vi "CMD_GETFLOATPOPUP.vi"(6 "Gantry in":refnum<class "Gantry.lvclass">, 8 "error in (no error)":errorcluster, 10 "Arguments":string[](array[string]), 11 "gScript Interpreter in":refnum<class "gScript Interpreter.lvclass">) -> (0 "error out":errorcluster, 3 "gScript Interpreter out":refnum<class "gScript Interpreter.lvclass">, 4 "Gantry out":refnum<class "Gantry.lvclass">)   [LabVIEW 2022 SP3, in "gScript Interpreter.lvclass"]
uses:
  gScript Interpreter.lvclass
  gScript Interpreter.lvclass/gScript Interpreter.ctl
  Shared Components/Gantry Class/Gantry.lvclass
panel:
  out "Message":string
  in  "Input":dbl format="%#g"
  in  "OK":bool caption="OK1"
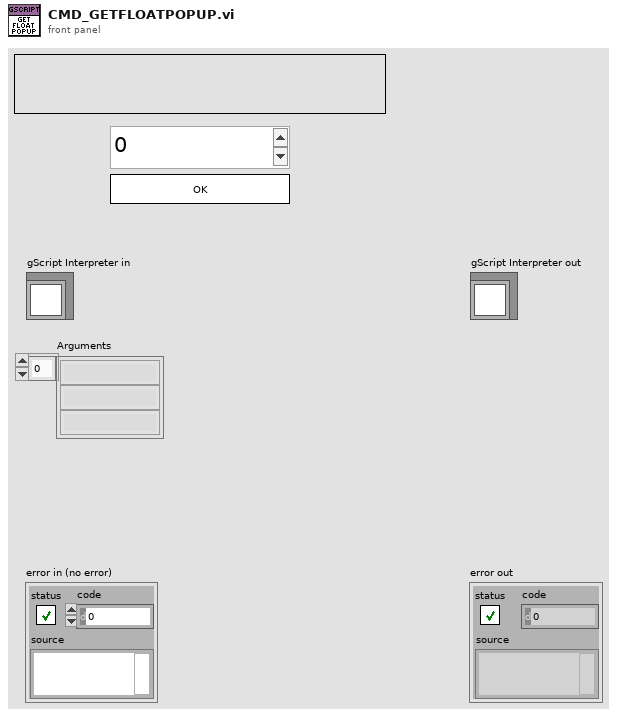
[diagram p1: front panel]
types:
  T1 = typedef "Memory Cell.ctl" = cluster{"type":T2, "x":dbl, "y":dbl, "z":dbl, "w":dbl}
  T2 = typedef "Memory Cell Type Enum.ctl" = enum16{"integer", "float", "vector", "rotation"}
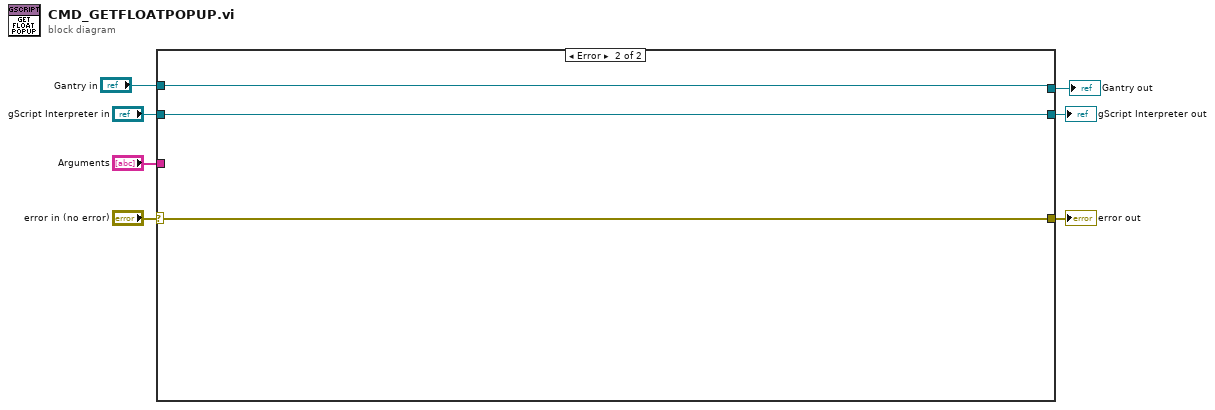
[diagram p0: block diagram]
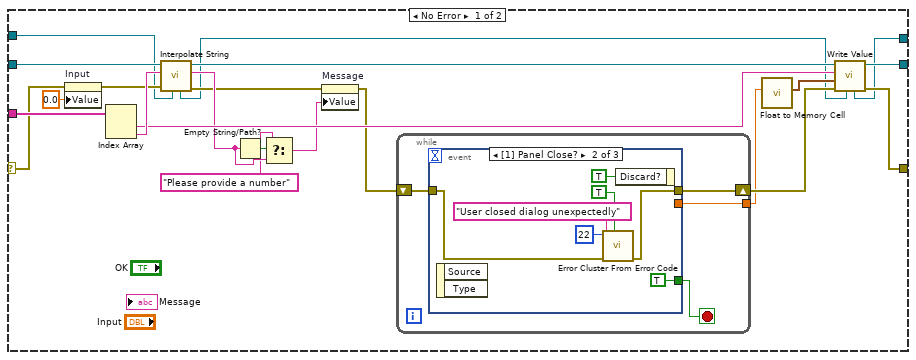
[diagram p2: hidden frame]
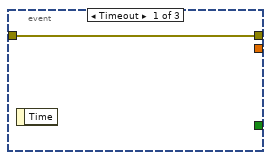
[diagram p3: hidden frame]
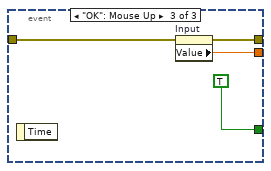
[diagram p4: hidden frame]
diagram:
  n1 = case shown="Error" "error in (no error)" {
    selector: "error in (no error)" -> [w13 w48]
    tunnel: [w25 w48] -> w6
    tunnel: [w24 w47] -> w4
    tunnel: "gScript Interpreter in" -> [w28 w47]
    tunnel: "Arguments" -> [w29 _]
    tunnel: "Gantry in" -> [w10 w46]
    tunnel: [w8 w46] -> w1
    frame No Error {
      n2 = property on="Input" class="DigNum (strict)"(error in=w13, "Value"=0.0 ("Input")) -> (error out=w12:errorcluster)  [unwired: 1 in, 1 out]
      n3 = Index Array(array=w29) -> (element #1=w26:string, element #2=w27:string)  [unwired: 2 in]
      n4 = call-dynamic "Interpolate String.vi"("Gantry in"=w10, "error in (no error)"=w12, "Input String"=w27, "gScript Interpreter in"=w28) -> ("error out"=w18:errorcluster, "Output String"=w22:string, "gScript Interpreter out"=w19:refnum<class "gScript Interpreter.lvclass">, "Gantry out"=w9:refnum<class "Gantry.lvclass">)  [unwired: 4 in]
      n5 = Empty String/Path?(string/path=w22) -> (empty?=w23:bool)
      n6 = Select(t="Please provide a number", s=w23, f=w22) -> (s? t:f=w20:string)
      n7 = property on="Message" class="Str"(error in=w18, "Value"=w20) -> (error out=w17:errorcluster)  [unwired: 1 in, 1 out]
      n8 = while {
        shift-right: [w31] -> w16
        shift-left: w17 -> [w32]
        tunnel: [w30] -> w15
        stop <- w33 stop-if-true
        n9 = event shown="[1] Panel Close?" {
          selector: _ -> [_ _ _]
          dyn-events: _ -> [_ _ _]
          timeout: _ -> [_ _ _]
          tunnel: [_ TRUE TRUE] -> w33
          tunnel: w32 -> [w34 w38 w44]
          tunnel: [w34 w37 w43] -> w31
          tunnel: [_ _ w42] -> w30
          event Timeout {
            n10 = event-data() -> ()  [unwired: 1 in, 1 out]
          }
          event Panel Close? {
            n11 = event-data() -> ()  [unwired: 1 in, 2 out]
            n12 = call <vilib>:"Error Cluster From Error Code.vi"("show call chain? (False)"=TRUE, "error in (no error)"=w38, "error message (\"\")"="User closed dialog unexpectedly" ("error message (\"\")"), "error code (0)"=22) -> ("error out"=w37:errorcluster)  [unwired: 5 in]
            n13 = event-data("Discard?"=TRUE) -> ()  [unwired: 1 in, 1 out]
          }
          event "OK": Mouse Up {
            n14 = event-data() -> ()  [unwired: 1 in, 1 out]
            n15 = property on="Input" class="DigNum (strict)"(error in=w44) -> (error out=w43:errorcluster, "Value"=w42:dbl)  [unwired: 1 in, 1 out]
          }
        }
      }
      n16 = call "Float to Memory Cell.vi"("Float in"=w15) -> ("Memory Cell"=w14:T1)  [unwired: 10 in]
      n17 = call-dynamic "Write Value.vi"("Gantry in"=w9, "error in (no error)"=w16, "Value"=w14, "Address"=w26, "gScript Interpreter in"=w19) -> ("error out"=w25:errorcluster, "gScript Interpreter out"=w24:refnum<class "gScript Interpreter.lvclass">, "Gantry out"=w8:refnum<class "Gantry.lvclass">)  [unwired: 4 in]
    }
    frame Error {
    }
  }
  "error out" <- w6
  "gScript Interpreter out" <- w4
  "Gantry out" <- w1
